vi "solar_voy Set Bits (COSMOS).vi"(4 "LabVIEW Flattened Value":string, 6 "Bit Element Size (Array only)":i32, 7 "ENDIAN":enum8{"BIG", "LITTLE"}(ring), 8 "COSMOS TYPE":T1, 9 "Bit Size":i32, 10 "Bit Offset":i32, 11 "Padded COSMOS Data in":string) -> (1 "LV value size truncated?":bool, 2 "Bit Offset Past Value":i32, 3 "COSMOS Data out":string)   [LabVIEW 2018]
doc: "This packs the bits in the COSMOS Data. The COSMOS Data string must be padded."
uses:
  solar_voy_def/solar_voy_def_ctl ITEM TYPE.ctl
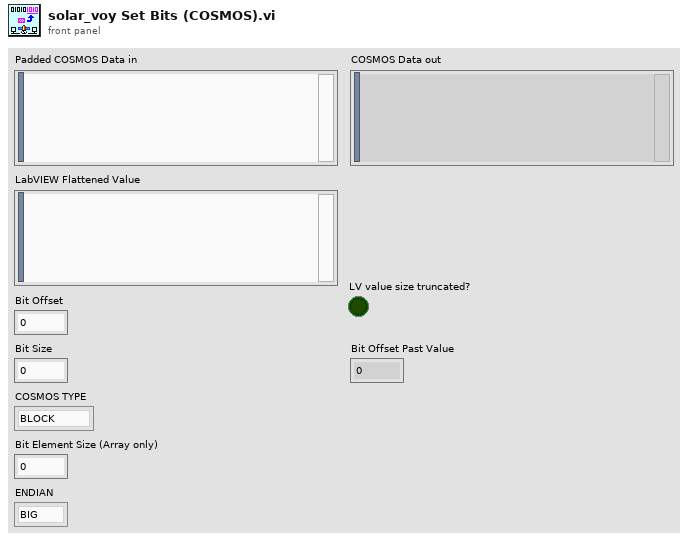
[diagram p1: front panel]
types:
  T1 = typedef "solar_voy_def_ctl ITEM TYPE.ctl" = enum8{"BLOCK", "INT", "UINT", "FLOAT", "STRING"}
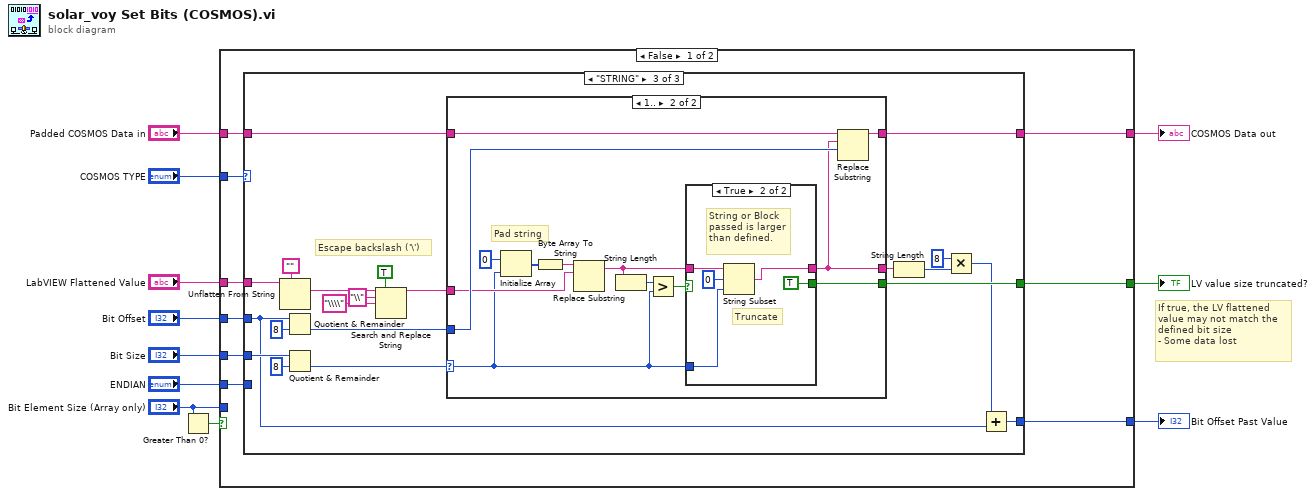
[diagram p0: block diagram]
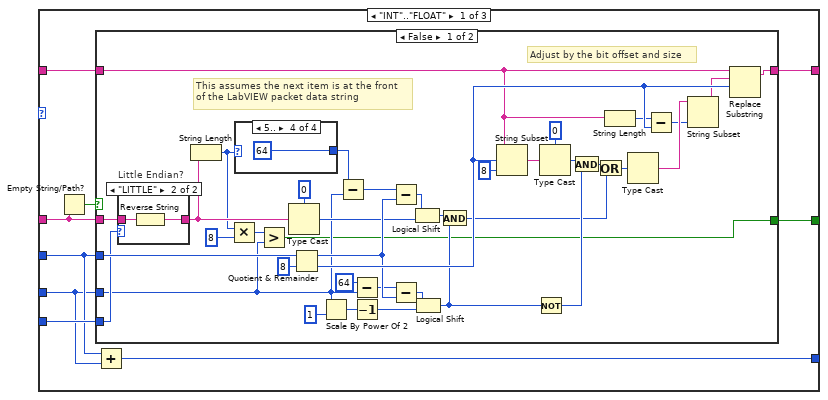
[diagram p2: hidden frame]
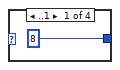
[diagram p4: hidden frame]
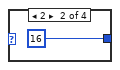
[diagram p5: hidden frame]
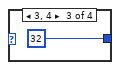
[diagram p6: hidden frame]
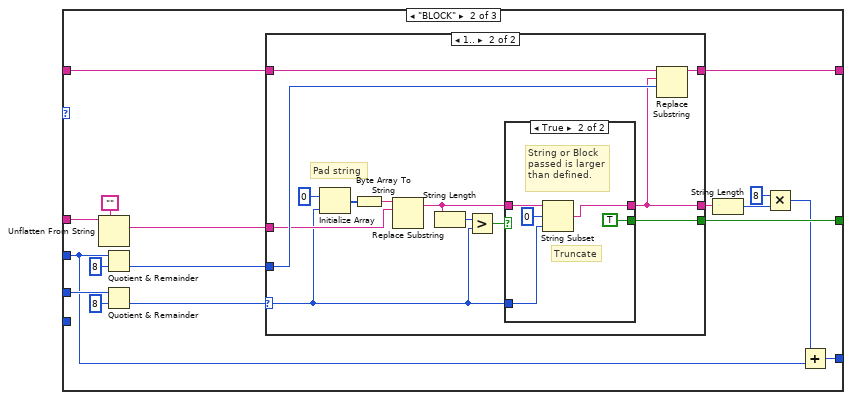
[diagram p8: hidden frame]
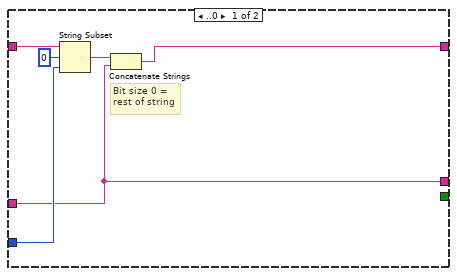
[diagram p9: hidden frame]
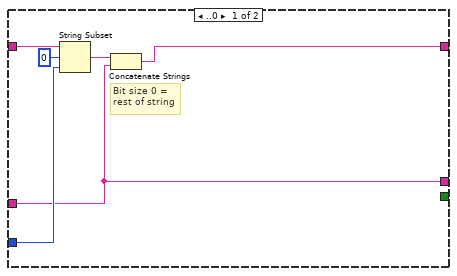
[diagram p11: hidden frame]
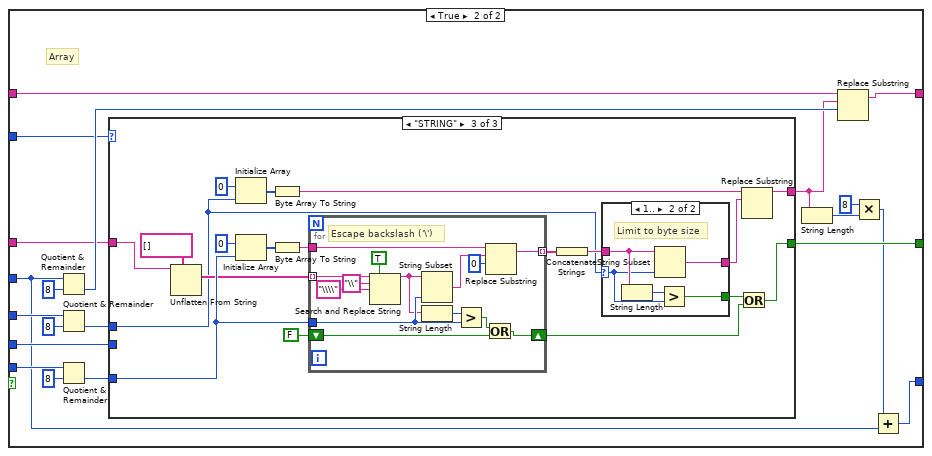
[diagram p13: hidden frame]
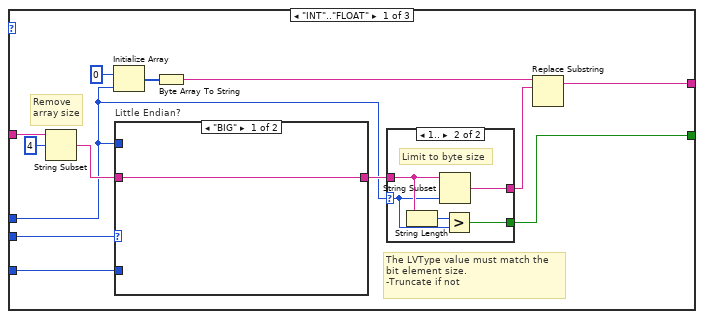
[diagram p14: hidden frame]
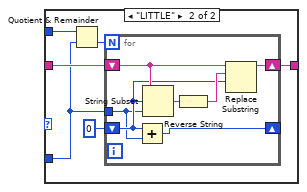
[diagram p16: hidden frame]
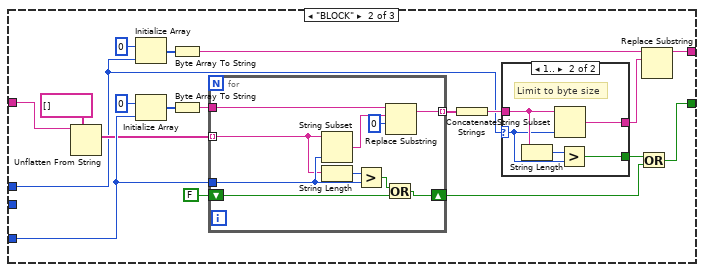
[diagram p17: hidden frame]
diagram:
  # "If true, the LV flattened\nvalue may not match the\ndefined bit size\n- Some data lost"
  n1 = Greater Than 0?(x="Bit Element Size (Array only)") -> (x > 0?=w1:bool)
  n2 = case shown="False" w1 {
    tunnel: "Padded COSMOS Data in" -> [w20 w178]
    tunnel: [w19 w174] -> w10
    tunnel: "Bit Offset" -> [w18 w167]
    tunnel: "COSMOS TYPE" -> [w17 w175]
    tunnel: "Bit Size" -> [w16 w172]
    tunnel: "ENDIAN" -> [w15 w177]
    tunnel: "LabVIEW Flattened Value" -> [w14 w176]
    tunnel: "Bit Element Size (Array only)" -> [_ w173]
    tunnel: [w13 w171] -> w4
    tunnel: [w12 w166] -> w3
    frame False {
      n3 = case shown="\"STRING\"" w17 {
        tunnel: w14 -> [w26 w85 w131]
        tunnel: [w28 w92 w138] -> w19
        tunnel: w20 -> [w27 w93 w139]
        tunnel: w16 -> [w23 w90 w136]
        tunnel: w18 -> [w24 w82 w129]
        tunnel: w15 -> [w25 _ _]
        tunnel: [w21 w83 w130] -> w13
        tunnel: [w22 w81 w128] -> w12
        frame "INT".."FLOAT" {
          n4 = Empty String/Path?(string/path=w26) -> (empty?=w29:bool)
          n5 = case shown="False" w29 {
            tunnel: w27 -> [w41 w76]
            tunnel: [w40 w76] -> w28
            tunnel: w24 -> [w39 _]
            tunnel: w26 -> [w38 _]
            tunnel: w23 -> [w31 _]
            tunnel: w25 -> [w35 _]
            tunnel: [w30 _] -> w21
            frame False {
              # "Adjust by the bit offset and size"
              # "This assumes the next item is at the front\nof the LabVIEW packet data string"
              n6 = case "Little Endian?" shown="\"LITTLE\"" w35 {
                tunnel: w38 -> [w69 w71]
                tunnel: [w69 w70] -> w36
                frame "BIG" {
                }
                frame "LITTLE" {
                  n7 = Reverse String(1:w71) -> (0:w70:string)
                }
              }
              n8 = String Length(string=w36) -> (length=w34:i32)
              n9 = Multiply(x=w34, y=8) -> (x*y=w32:i32)
              n10 = case shown="5.." w34 {
                tunnel: [8 16 32 64] -> w47
                frame ..1 {
                }
                frame 2 {
                }
                frame 3, 4 {
                }
                frame 5.. {
                }
              }
              n11 = Greater?(x=w32, y=w31) -> (0:w30:bool)
              n12 = Type Cast(type=u64 0, x=w36) -> (*(type *) &x=w65:u64)
              n13 = Quotient & Remainder(x=w39, y=8) -> (x-y*floor(x/y)=w66:i32, floor(x/y)=w67:i32)
              n14 = Scale By Power Of 2(n=w31, x=u64 1) -> (x*2^n=w54:u64)
              n15 = Subtract(x=w47, y=w31) -> (x-y=w46:i32)
              n16 = Subtract(x=64, y=w31) -> (x-y=w43:i32)
              n17 = Decrement(x=w54) -> (x-1=w55:u64)
              n18 = Subtract(x=w46, y=w66) -> (x-y=w45:i32)
              n19 = Subtract(x=w43, y=w66) -> (x-y=w42:i32)
              n20 = Logical Shift(y=w45, x=w65) -> (x << y=w60:u64)
              n21 = Logical Shift(y=w42, x=w55) -> (x << y=w61:u64)
              n22 = And(x=w60, y=w61) -> (x .and. y?=w37:u64)
              n23 = String Subset(string=w41, offset (0)=w67, length (rest)=8 ("length (rest)")) -> (substring=w52:string)
              n24 = Not(x=w61) -> (.not. x?=w57:u64)
              n25 = Type Cast(type=u64 0, x=w52) -> (*(type *) &x=w56:u64)
              n26 = And(x=w56, y=w57) -> (x .and. y?=w58:u64)
              n27 = Or(x=w58, y=w37) -> (x .or. y?=w59:u64)
              n28 = String Length(string=w41) -> (length=w49:i32)
              n29 = Type Cast(x=w59) -> (*(type *) &x=w62:string)  [unwired: 1 in]
              n30 = Subtract(x=w49, y=w67) -> (x-y=w48:i32)
              n31 = String Subset(string=w62, length (rest)=w48) -> (substring=w63:string)  [unwired: 1 in]
              n32 = Replace Substring(3:w67, 4:w63, 5:w41) -> (1:w40:string)  [unwired: 2 out]
            }
            frame True {
            }
          }
          n33 = Add(x=w24, y=w23) -> (x+y=w22:i32)
        }
        frame "BLOCK" {
          n34 = Unflatten From String(type="", binary string=w85) -> (value=w84:string)  [unwired: 3 in, 2 out]
          n35 = Quotient & Remainder(x=w82, y=8) -> (floor(x/y)=w88:i32)  [unwired: 1 out]
          n36 = Quotient & Remainder(x=w90, y=8) -> (floor(x/y)=w87:i32)  [unwired: 1 out]
          n37 = case shown="1.." w87 {
            selector: w87 -> [_ w103]
            tunnel: w93 -> [w99 w109]
            tunnel: [w95 w108] -> w92
            tunnel: w88 -> [w98 w107]
            tunnel: w84 -> [w94 w106]
            tunnel: [_ w101] -> w83
            tunnel: [w94 w100] -> w77
            frame ..0 {
              # "Bit size 0 =\nrest of string"
              n38 = String Subset(string=w99, offset (0)=0, length (rest)=w98) -> (substring=w96:string)
              n39 = Concatenate Strings(w96, w94) -> (w95:string)
            }
            frame 1.. {
              # "Pad string"
              n40 = Initialize Array(u8 0, w103) -> (w111:u8[])
              n41 = Byte Array To String(unsigned byte array=w111) -> (string=w110:string)
              n42 = Replace Substring(4:w106, 5:w110) -> (1:w104:string)  [unwired: 3 out]
              n43 = String Length(string=w104) -> (length=w105:i32)
              n44 = Greater?(x=w105, y=w103) -> (0:w102:bool)
              n45 = case shown="True" w102 {
                tunnel: w104 -> [w113 w118]
                tunnel: [w113 w115] -> w100
                tunnel: w103 -> [_ w116]
                tunnel: [_ TRUE] -> w101
                frame False {
                }
                frame True {
                  # "Truncate"
                  # "String or Block\npassed is larger\nthan defined."
                  n46 = String Subset(string=w118, offset (0)=0, length (rest)=w116) -> (substring=w115:string)
                }
              }
              n47 = Replace Substring(3:w107, 4:w100, 5:w109) -> (1:w108:string)  [unwired: 2 out]
            }
          }
          n48 = String Length(string=w77) -> (length=w79:i32)
          n49 = Multiply(x=8, y=w79) -> (x*y=w78:i32)
          n50 = Add(x=w78, y=w82) -> (x+y=w81:i32)
        }
        frame "STRING" {
          # "Escape backslash ('\\')"
          n51 = Unflatten From String(type="", binary string=w131) -> (value=w120:string)  [unwired: 3 in, 2 out]
          n52 = Quotient & Remainder(x=w129, y=8) -> (floor(x/y)=w134:i32)  [unwired: 1 out]
          n53 = Quotient & Remainder(x=w136, y=8) -> (floor(x/y)=w133:i32)  [unwired: 1 out]
          n54 = Search and Replace String(replace all?=TRUE ("replace all? (F)"), input string=w120, search string="\\", replace string="\\\\" ("search string")) -> (result string=w119:string)  [unwired: 4 in, 3 out]
          n55 = case shown="1.." w133 {
            selector: w133 -> [_ w149]
            tunnel: w139 -> [w145 w155]
            tunnel: [w141 w154] -> w138
            tunnel: w134 -> [w144 w153]
            tunnel: w119 -> [w140 w152]
            tunnel: [_ w147] -> w130
            tunnel: [w140 w146] -> w124
            frame ..0 {
              # "Bit size 0 =\nrest of string"
              n56 = String Subset(string=w145, offset (0)=0, length (rest)=w144) -> (substring=w142:string)
              n57 = Concatenate Strings(w142, w140) -> (w141:string)
            }
            frame 1.. {
              # "Pad string"
              n58 = Initialize Array(u8 0, w149) -> (w157:u8[])
              n59 = Byte Array To String(unsigned byte array=w157) -> (string=w156:string)
              n60 = Replace Substring(4:w152, 5:w156) -> (1:w150:string)  [unwired: 3 out]
              n61 = String Length(string=w150) -> (length=w151:i32)
              n62 = Greater?(x=w151, y=w149) -> (0:w148:bool)
              n63 = case shown="True" w148 {
                tunnel: w150 -> [w159 w164]
                tunnel: [w159 w161] -> w146
                tunnel: w149 -> [_ w162]
                tunnel: [_ TRUE] -> w147
                frame False {
                }
                frame True {
                  # "Truncate"
                  # "String or Block\npassed is larger\nthan defined."
                  n64 = String Subset(string=w164, offset (0)=0, length (rest)=w162) -> (substring=w161:string)
                }
              }
              n65 = Replace Substring(3:w153, 4:w146, 5:w155) -> (1:w154:string)  [unwired: 2 out]
            }
          }
          n66 = String Length(string=w124) -> (length=w126:i32)
          n67 = Multiply(x=8, y=w126) -> (x*y=w125:i32)
          n68 = Add(x=w125, y=w129) -> (x+y=w128:i32)
        }
      }
    }
    frame True {
      # "Array"
      n69 = Quotient & Remainder(x=w167, y=8) -> (floor(x/y)=w183:i32)  [unwired: 1 out]
      n70 = Quotient & Remainder(x=w172, y=8) -> (floor(x/y)=w181:i32)  [unwired: 1 out]
      n71 = Quotient & Remainder(x=w173, y=8) -> (floor(x/y)=w179:i32)  [unwired: 1 out]
      n72 = case shown="\"STRING\"" w175 {
        tunnel: w176 -> [w196 w236 w271]
        tunnel: [w192 w224 w259] -> w170
        tunnel: w181 -> [w186 w221 w256]
        tunnel: w177 -> [w191 _ _]
        tunnel: w179 -> [w189 w235 w270]
        tunnel: [w185 w219 w254] -> w171
        frame "INT".."FLOAT" {
          # "The LVType value must match the\nbit element size.\n-Truncate if not"
          # "Remove \narray size"
          n73 = String Subset(string=w196, offset (0)=4) -> (substring=w190:string)  [unwired: 1 in]
          n74 = Initialize Array(u8 0, w186) -> (w194:u8[])
          n75 = case "Little Endian?" shown="\"BIG\"" w191 {
            tunnel: w190 -> [w204 w209]
            tunnel: [w204 w208] -> w187
            tunnel: w189 -> [_ w207]
            tunnel: w186 -> [_ w206]
            frame "BIG" {
            }
            frame "LITTLE" {
              n76 = Quotient & Remainder(x=w206, y=w207) -> (floor(x/y)=w210:i32)  [unwired: 1 out]
              n77 = for {
                N: w210 -> [_]
                shift-right: [w214] -> w208
                shift-left: w209 -> [w215]
                shift-right: [w217] -> _
                shift-left: 0 -> [w212]
                tunnel: w207 -> [w211]
                n78 = Add(x=w212, y=w211) -> (x+y=w217:i32)
                n79 = String Subset(string=w215, offset (0)=w212, length (rest)=w211) -> (substring=w216:string)
                n80 = Reverse String(1:w216) -> (0:w213:string)
                n81 = Replace Substring(3:w212, 4:w213, 5:w215) -> (1:w214:string)  [unwired: 1 in, 1 out]
              }
            }
          }
          n82 = Byte Array To String(unsigned byte array=w194) -> (string=w193:string)
          n83 = case shown="1.." w186 {
            selector: w186 -> [_ w200]
            tunnel: [w198 w203] -> w188
            tunnel: w187 -> [w198 w202]
            tunnel: [_ w199] -> w185
            frame ..0 {
              # "Rest"
            }
            frame 1.. {
              # "Limit to byte size"
              n84 = String Length(string=w202) -> (length=w201:i32)
              n85 = String Subset(string=w202, length (rest)=w200) -> (substring=w203:string)  [unwired: 1 in]
              n86 = Greater?(x=w201, y=w200) -> (0:w199:bool)
            }
          }
          n87 = Replace Substring(4:w188, 5:w193) -> (1:w192:string)  [unwired: 3 out]
        }
        frame "BLOCK" {
          n88 = Unflatten From String(type=string[] [], binary string=w236) -> (value=w234:string[])  [unwired: 3 in, 2 out]
          n89 = Initialize Array(u8 0, w221) -> (w233:u8[])
          n90 = Initialize Array(u8 0, w235) -> (w230:u8[])
          n91 = Byte Array To String(unsigned byte array=w233) -> (string=w226:string)
          n92 = Byte Array To String(unsigned byte array=w230) -> (string=w229:string)
          n93 = for {
            tunnel: w234 -> [w245] mode=indexing
            tunnel: w235 -> [w246]
            shift-right: [w249] -> w218
            shift-left: FALSE -> [w250]
            tunnel: w229 -> [w248]
            tunnel: [w243] -> w225 mode=indexing
            n94 = String Subset(string=w245, length (rest)=w246) -> (substring=w244:string)  [unwired: 1 in]
            n95 = String Length(string=w245) -> (length=w252:i32)
            n96 = Greater?(x=w252, y=w246) -> (0:w251:bool)
            n97 = Or(x=w251, y=w250) -> (x .or. y?=w249:bool)
            n98 = Replace Substring(3:0 ("offset (0)"), 4:w244, 5:w248) -> (1:w243:string)  [unwired: 2 out]
          }
          n99 = Concatenate Strings(w225) -> (w223:string)
          n100 = case shown="1.." w221 {
            selector: w221 -> [_ w239]
            tunnel: [w237 w242] -> w222
            tunnel: w223 -> [w237 w241]
            tunnel: [_ w238] -> w220
            frame ..0 {
              # "Rest"
            }
            frame 1.. {
              # "Limit to byte size"
              n101 = String Length(string=w241) -> (length=w240:i32)
              n102 = String Subset(string=w241, length (rest)=w239) -> (substring=w242:string)  [unwired: 1 in]
              n103 = Greater?(x=w240, y=w239) -> (0:w238:bool)
            }
          }
          n104 = Or(x=w220, y=w218) -> (x .or. y?=w219:bool)
          n105 = Replace Substring(4:w222, 5:w226) -> (1:w224:string)  [unwired: 3 out]
        }
        frame "STRING" {
          n106 = Unflatten From String(type=string[] [], binary string=w271) -> (value=w269:string[])  [unwired: 3 in, 2 out]
          n107 = Initialize Array(u8 0, w256) -> (w268:u8[])
          n108 = Initialize Array(u8 0, w270) -> (w265:u8[])
          n109 = Byte Array To String(unsigned byte array=w268) -> (string=w261:string)
          n110 = Byte Array To String(unsigned byte array=w265) -> (string=w264:string)
          n111 = for {
            tunnel: w269 -> [w279] mode=indexing
            tunnel: w270 -> [w285]
            shift-right: [w288] -> w253
            shift-left: FALSE -> [w289]
            tunnel: w264 -> [w287]
            tunnel: [w283] -> w260 mode=indexing
            # "Escape backslash ('\\')"
            n112 = Search and Replace String(replace all?=TRUE ("replace all? (F)"), input string=w279, search string="\\", replace string="\\\\" ("search string")) -> (result string=w278:string)  [unwired: 4 in, 3 out]
            n113 = String Subset(string=w278, length (rest)=w285) -> (substring=w284:string)  [unwired: 1 in]
            n114 = String Length(string=w278) -> (length=w291:i32)
            n115 = Greater?(x=w291, y=w285) -> (0:w290:bool)
            n116 = Or(x=w290, y=w289) -> (x .or. y?=w288:bool)
            n117 = Replace Substring(3:0 ("offset (0)"), 4:w284, 5:w287) -> (1:w283:string)  [unwired: 2 out]
          }
          n118 = Concatenate Strings(w260) -> (w258:string)
          n119 = case shown="1.." w256 {
            selector: w256 -> [_ w274]
            tunnel: [w272 w277] -> w257
            tunnel: w258 -> [w272 w276]
            tunnel: [_ w273] -> w255
            frame ..0 {
              # "Rest"
            }
            frame 1.. {
              # "Limit to byte size"
              n120 = String Length(string=w276) -> (length=w275:i32)
              n121 = String Subset(string=w276, length (rest)=w274) -> (substring=w277:string)  [unwired: 1 in]
              n122 = Greater?(x=w275, y=w274) -> (0:w273:bool)
            }
          }
          n123 = Or(x=w255, y=w253) -> (x .or. y?=w254:bool)
          n124 = Replace Substring(4:w257, 5:w261) -> (1:w259:string)  [unwired: 3 out]
        }
      }
      n125 = String Length(string=w170) -> (length=w169:i32)
      n126 = Replace Substring(3:w183, 4:w170, 5:w178) -> (1:w174:string)  [unwired: 2 out]
      n127 = Multiply(x=8, y=w169) -> (x*y=w165:i32)
      n128 = Add(x=w165, y=w167) -> (x+y=w166:i32)
    }
  }
  "COSMOS Data out" <- w10
  "Bit Offset Past Value" <- w3
  "LV value size truncated?" <- w4
